vi "Get Actor Handles.vi"() -> (2 "Actor Handles":refnum<class "Protected Actor Handle.lvclass">[](array[class]))   [LabVIEW 2020, in "AF Debug.lvlib"]
doc: "This VI returns an array of handles for currently running actors to use in a debugging tool. Actors are wrapped in handles to limit a debugger's ability to interfere with the operation of the actors and to protect the debugger from actors stopping unexpectedly."
uses:
  AF Debug.lvlib
  Registration Mode.ctl
  Protected Actor Handle/Protected Actor Handle.lvclass
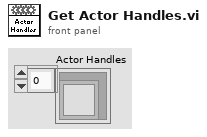
[diagram p1: front panel]
types:
  T1 = typedef "AF Debug.lvlib/Registration Mode.ctl" = enum16{"Register Actor", "Get ID", "Get Enqueuer", "Deregister Actor", "Get Update Event", "Get All Actors"}
  T2 = typedef "AF Debug.lvlib/This Actor.ctl" = cluster{"Enqueuer":refnum<class "Message Enqueuer.lvclass">, "ID":string, "Alias":string, "Actor Core Name":string, "Details":cluster{"Qualified Name":string, "Caller ID":string}}
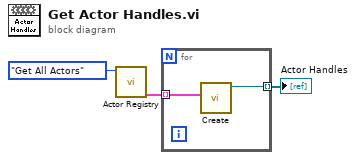
[diagram p0: block diagram]
diagram:
  n1 = call "Actor Registry.vi"("Action"=Registration_Mode."Get All Actors") -> ("All Actors"=w2:T2[])  [unwired: 6 in, 4 out]
  n2 = for {
    tunnel: w2 -> [w5] mode=indexing
    tunnel: [w4] -> w1 mode=indexing
    n3 = call "Create.vi"("This Actor"=w5) -> ("Protected Actor Handle out"=w4:refnum<class "Protected Actor Handle.lvclass">)  [unwired: 9 in, 1 out]
  }
  "Actor Handles" <- w1
